vi "Problem 9 - Special Pythagorean triplet.vi"() -> (3 "Answer":i32)   [LabVIEW 2021, in "Project Euler.lvlib"]
uses:
  Project Euler.lvlib
  cluster-double.ctl
  cluster-triplet.ctl
  Utilities/Named Counters/Named Counters.lvlib
  Utilities/Named Timers/Named Timers.lvlib
panel:
  out "Execution time (ms)":u32
  out "Computational complexity counter":i32
  out "Pythagorean triplets whose sum is equal to desired":T1[](array[typedef])
  out "(a,b)":T2
  in  "desired sum of triplet (dflt=1000)":i32=1000
  # "Development\nControls or indicators that are useful for development or testing, but which are not outputs of the VI."
  # "Input\nInputs to the VI"
  # "Output\nOutputs of the VI"
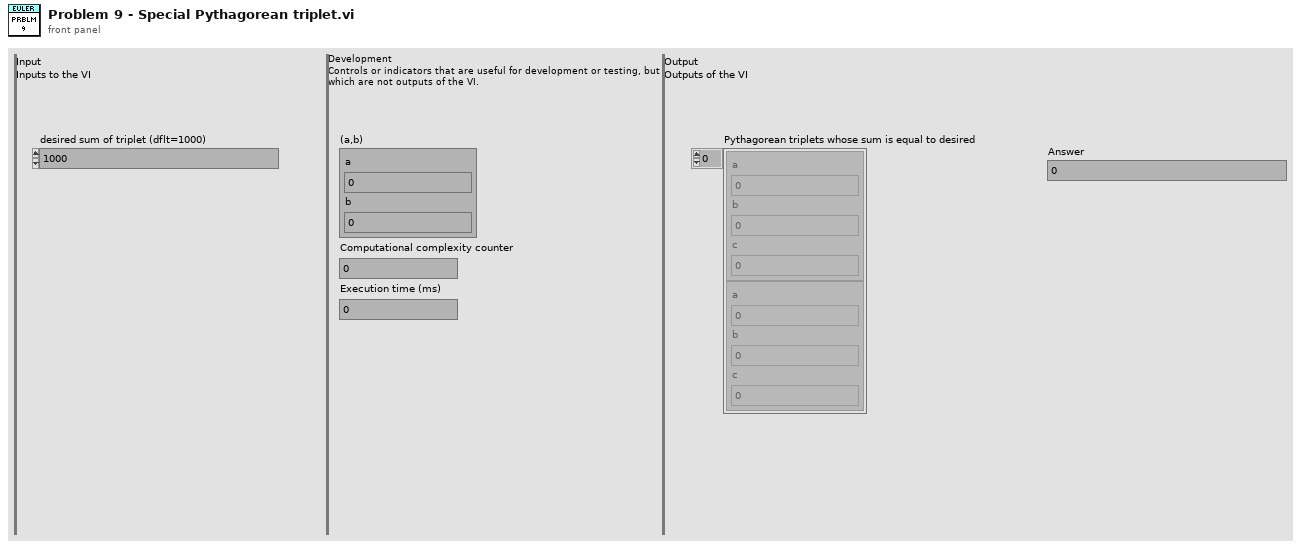
[diagram p1: front panel]
types:
  T1 = typedef "Project Euler.lvlib/cluster-triplet.ctl" = cluster{"a":i32, "b":i32, "c":i32}
  T2 = typedef "Project Euler.lvlib/cluster-double.ctl" = cluster{"a":i32, "b":i32}
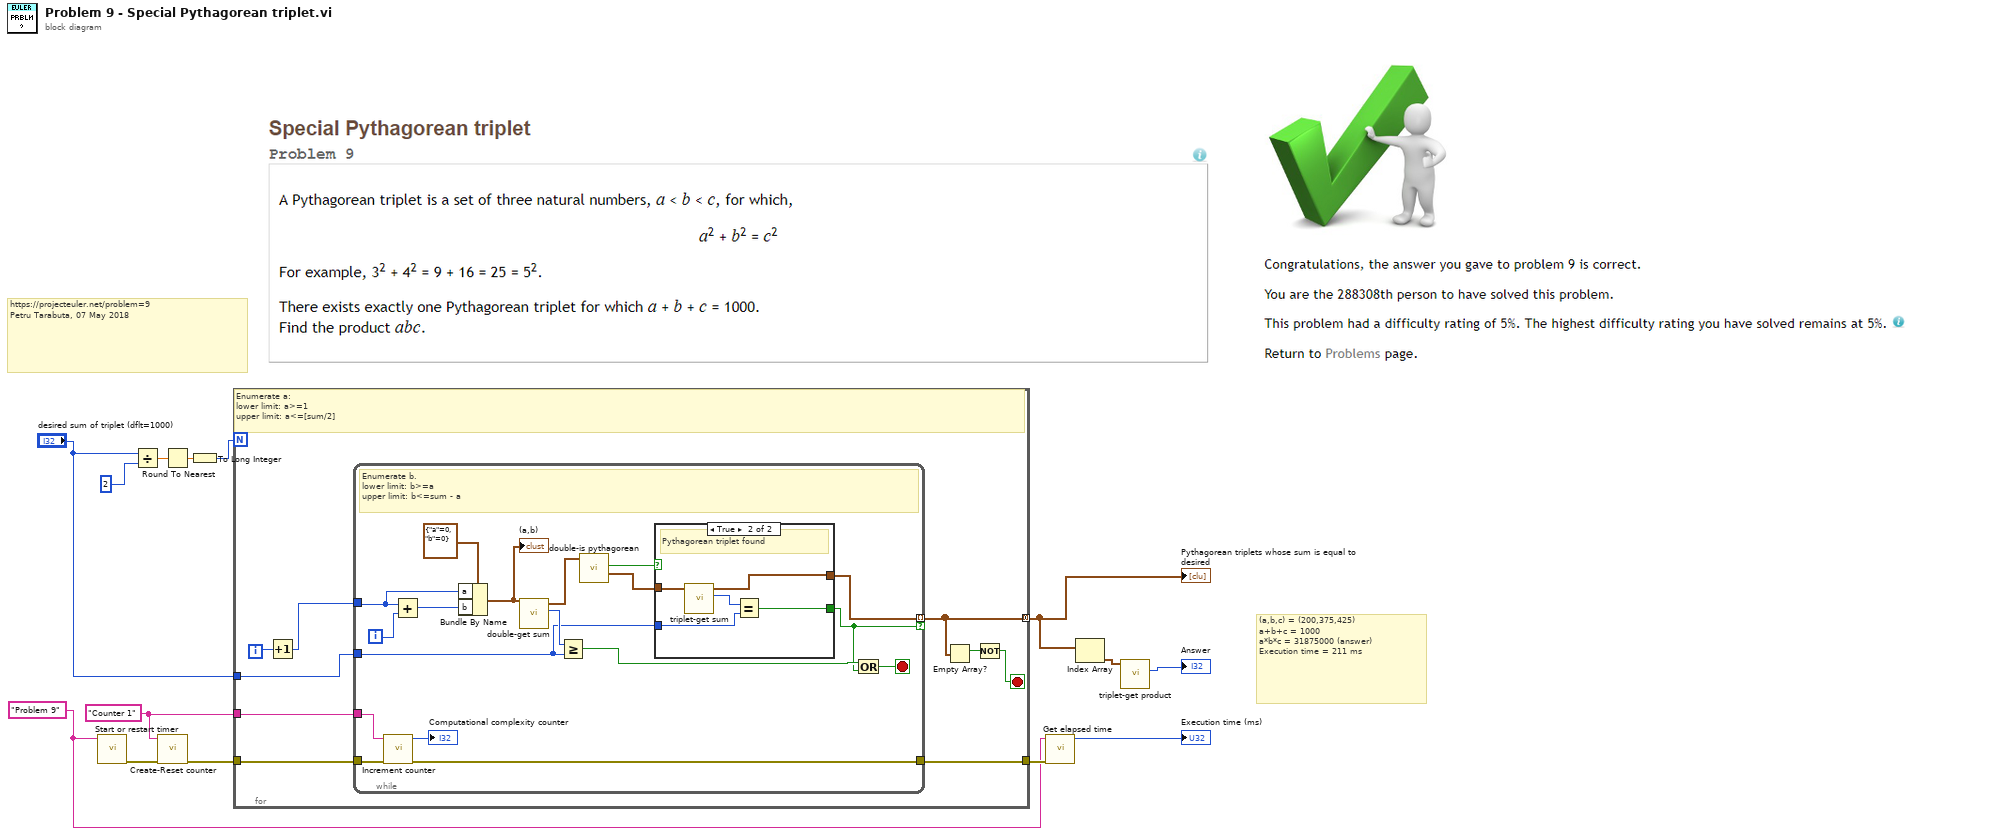
[diagram p0: block diagram]
diagram:
  w5 = "Problem 9" ("Counter name (dflt=blank)")
  w8 = "Counter 1" ("Counter name (dflt=blank)")
  # "(a,b,c) = (200,375,425)\na+b+c = 1000\na*b*c = 31875000 (answer)\nExecution time = 211 ms"
  # "https://projecteuler.net/problem=9\nPetru Tarabuta, 07 May 2018"
  n1 = call "Start or restart timer.vi"("Timer name"=w5) -> ("error out"=w7:errorcluster)  [unwired: 10 in]
  n2 = Divide(x="desired sum of triplet (dflt=1000)", y=u32 2) -> (x/y=w13:dbl)
  n3 = call "Create-Reset counter.vi"("error in (no error)"=w7, "Counter name (dflt=blank)"=w8) -> ("error out"=w9:errorcluster)  [unwired: 9 in]
  n4 = Round To Nearest(number=w13) -> (nearest integer value=w12:dbl)
  n5 = To Long Integer(number=w12) -> (32bit integer=w11:i32)
  n6 = for {
    N: w11 -> [_]
    tunnel: "desired sum of triplet (dflt=1000)" -> [w21]
    tunnel: [w17] -> w3 mode=concatenating
    tunnel: w9 -> [w19]
    tunnel: w8 -> [w20]
    tunnel: [w18] -> w6
    i -> [w23]
    stop <- w15 stop-if-true
    # "Enumerate a: \nlower limit: a>=1\nupper limit: a<=[sum/2]"
    n7 = Increment(x=w23) -> (x+1=w22:i32)
    n8 = while {
      tunnel: w22 -> [w40]
      tunnel: w21 -> [w32]
      tunnel: [w31] -> w17 mode=indexing if=w25
      tunnel: w20 -> [w30]
      tunnel: w19 -> [w29]
      tunnel: [w28] -> w18
      i -> [w41]
      stop <- w24 stop-if-true
      # "Enumerate b.\nlower limit: b>=a\nupper limit: b<=sum - a"
      n9 = call "Increment counter.vi"("error in (no error)"=w29, "Counter name (dflt=blank)"=w30) -> ("error out"=w28:errorcluster, "Value (after increment)"=→"Computational complexity counter":i32)  [unwired: 8 in]
      n10 = Add(x=w40, y=w41) -> (x+y=w38:i32)
      n11 = Bundle By Name(cluster=T2 {"a"=0, "b"=0} ("(a, b)"), "a"=w40, "b"=w38) -> (w35:T2)
      "(a,b)" <- w35
      n12 = call "double-get sum.vi"("(a, b) in"=w35) -> ("sum = a+b"=w37:i32, "(a, b) out (duplicate)"=w36:T2)  [unwired: 8 in, 1 out]
      n13 = Greater Or Equal?(x=w37, y=w32) -> (x >= y?=w26:bool)
      n14 = call "double-is pythagorean.vi"("(a, b) in"=w36) -> ("Pythagorean triplet"=w33:T1, "T = this double is Pythagorean (a^2+b^2=c^2)"=w34:bool)  [unwired: 7 in, 2 out]
      n15 = case shown="True" w34 {
        tunnel: w33 -> [_ w46]
        tunnel: w32 -> [_ w44]
        tunnel: [_ w43] -> w25
        tunnel: [_ w42] -> w31
        frame False {
        }
        frame True {
          # "Pythagorean triplet found"
          n16 = call "triplet-get sum.vi"("(a, b, c) in"=w46) -> ("sum = a+b+c"=w45:i32, "(a, b, c) out (duplicate)"=w42:T1)  [unwired: 8 in, 1 out]
          n17 = Equal?(x=w45, y=w44) -> (x = y?=w43:bool)
        }
      }
      n18 = Or(x=w26, y=w25) -> (x .or. y?=w24:bool)
    }
    n19 = Empty Array?(array=w17) -> (empty?=w16:bool)
    n20 = Not(x=w16) -> (.not. x?=w15:bool)
  }
  "Pythagorean triplets whose sum is equal to desired" <- w3
  n21 = call "Get elapsed time.vi"("error in (no error)"=w6, "Timer name"=w5) -> ("Elapsed time (ms)"=→"Execution time (ms)":u32)  [unwired: 6 in, 3 out]
  n22 = Index Array(array=w3) -> (element=w2:T1)  [unwired: 1 in]
  n23 = call "triplet-get product.vi"("(a, b, c) in"=w2) -> ("product = a+b+c"=→"Answer":i32)  [unwired: 8 in, 2 out]
